vi "Read Joystick.vi"(8 "error in (no error)":errorcluster, 11 "XBoxController in":refnum<class "XBoxController.lvclass">) -> (0 "error out":errorcluster, 3 "XBoxController out":refnum<class "XBoxController.lvclass">)   [LabVIEW 2013, in "XBoxController.lvlib" / "XBoxController.lvclass"]
uses:
  XBoxController.lvclass
  XBoxController.lvclass/XBoxController.ctl
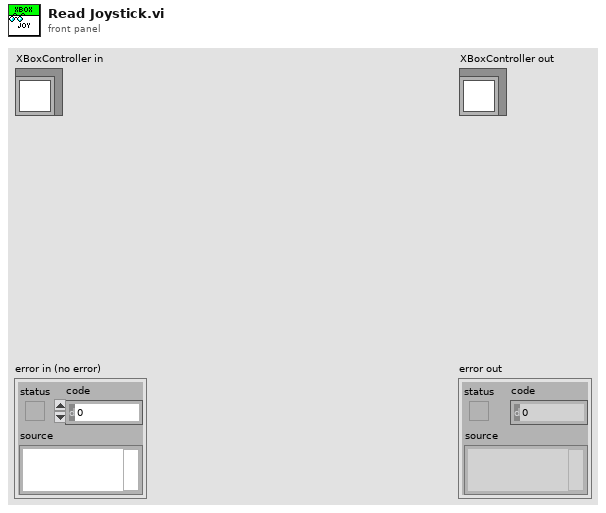
[diagram p1: front panel]
types:
  T1 = typedef "XBoxController.lvlib/XboxJoysticks.ctl" = cluster{"LeftJoystick":cluster{"Forward":dbl, "Right":dbl}, "RightJoystick":cluster{"Forward":dbl, "Right":dbl}}
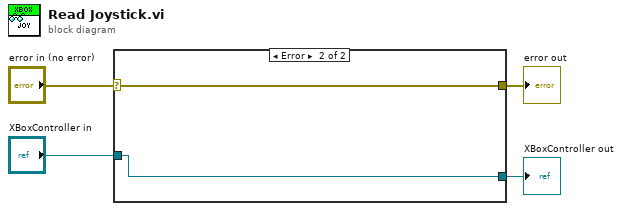
[diagram p0: block diagram]
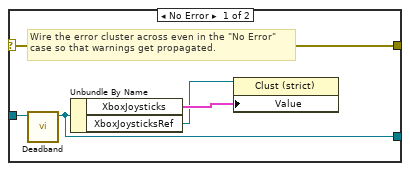
[diagram p2: hidden frame]
diagram:
  n1 = case shown="Error" "error in (no error)" {
    selector: "error in (no error)" -> [w9 w11]
    tunnel: [w9 w11] -> w3
    tunnel: "XBoxController in" -> [w8 w10]
    tunnel: [w7 w10] -> w1
    frame No Error {
      # "Wire the error cluster across even in the \"No Error\"\ncase so that warnings get propagated."
      n2 = call-dynamic "Deadband.vi"("XBoxController in"=w8) -> ("XBoxController out"=w7:refnum<class "XBoxController.lvclass">)  [unwired: 9 in, 1 out]
      n3 = Unbundle By Name(w7) -> ("XboxJoysticks"=w6:T1, "XboxJoysticksRef"=w5:refnum<vi>)
      n4 = property class="Clust (strict)"(reference=w5, "Value"=w6) -> ()  [unwired: 1 in, 2 out]
    }
    frame Error {
    }
  }
  "error out" <- w3
  "XBoxController out" <- w1
